vi "电导率_所有参数读取.vi"(8 "error in (no error)":errorcluster caption="错误输入（无错误）", 11 "MB session in":refnum<class "MB_Master.lvclass">) -> (0 "error out":errorcluster caption="错误输出", 2 "输出值":T1 {"电极型号标志" items=["NULL", "pH", "Cond", "DO", "Turb"]; "电极状态标志" items=["OK"]}, 3 "MB session out":refnum<class "MB_Master.lvclass">)   [LabVIEW 2016, in "斯坦道多参数.lvlib"]
uses:
  <vilib>/Plasmionique/MB Master/MB_Master/MB_Master.lvclass
  <vilib>/Plasmionique/MB Master/MB Master.lvlib
  <vilib>/ptbypt/NI_PtbyPt.lvlib
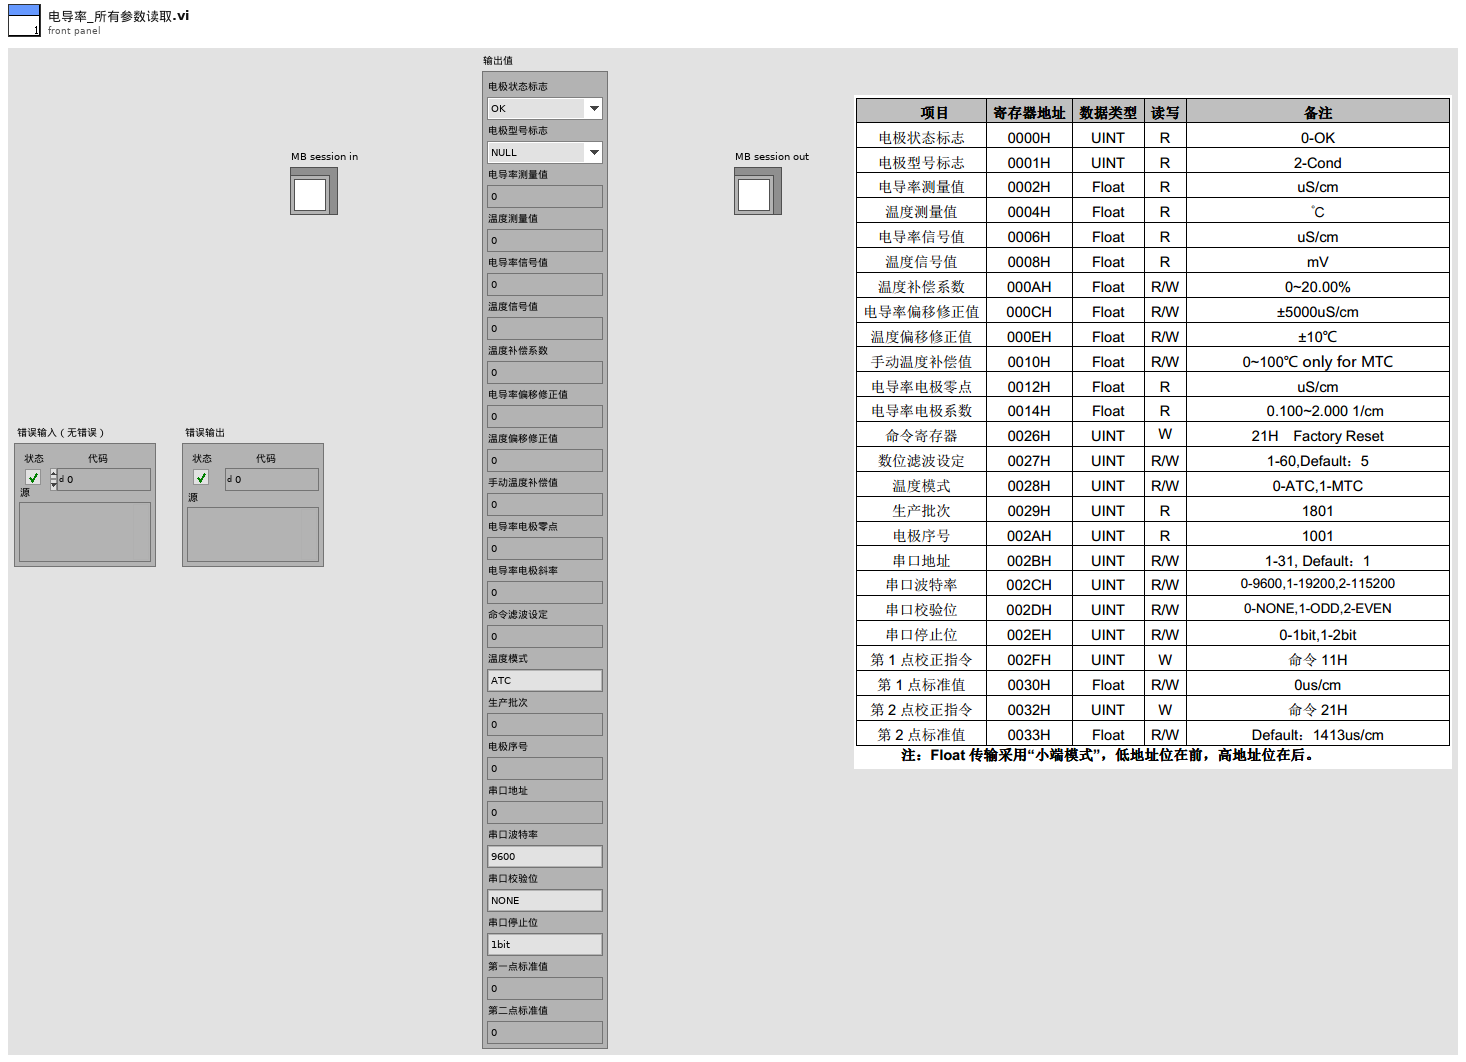
[diagram p1: front panel]
types:
  T1 = cluster{"电极状态标志":u16, "电极型号标志":u16, "电导率测量值":sgl, "温度测量值":sgl, "电导率信号值":sgl, "温度信号值":sgl, "温度补偿系数":sgl, "电导率偏移修正值":sgl, "温度偏移修正值":sgl, "手动温度补偿值":sgl, "电导率电极零点":sgl, "电导率电极斜率":sgl, "命令滤波设定":u16, "温度模式":enum16{"ATC", "MTC"}, "生产批次":u16, "电极序号":u16, "串口地址":u16, "串口波特率":enum16{"9600", "19200", "115200"}, "串口校验位":enum16{"NONE", "ODD", "EVEN"}, "串口停止位":enum16{"1bit", "2bit"}, "第一点标准值":sgl, "第二点标准值":sgl}
  T2 = cluster{u16, u16, "Filtered x":dbl, "数值":sgl, "数值":sgl, "数值":sgl, "数值":sgl, "数值":sgl, "数值":sgl, "数值":sgl, "数值":sgl, "数值":sgl, u16, u16, u16, u16, u16, u16, u16, u16, "数值":sgl, "数值":sgl}
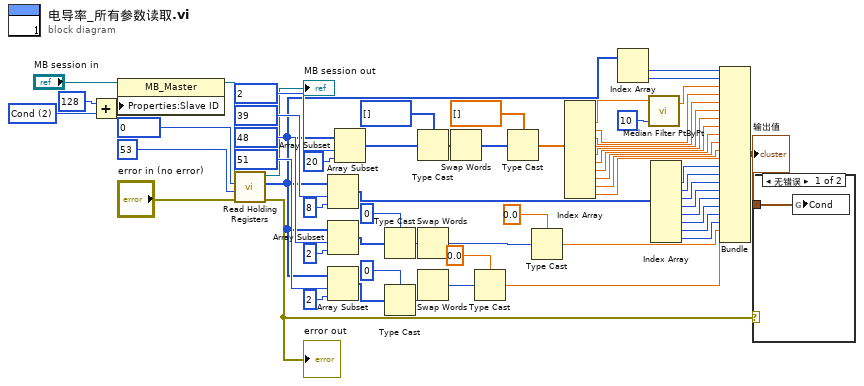
[diagram p0: block diagram]
diagram:
  w61 = u16 2 items=["NULL", "pH", "Cond", "DO", "Turb"] ("数值")
  n1 = Add(x=u16 128, y=w61) -> (x+y=w60:u16)
  n2 = property class="MB_Master"(reference="MB session in", "Properties:Slave ID"=w60) -> (reference out=w14:refnum<class "MB_Master.lvclass">)  [unwired: 1 in, 1 out]
  n3 = call <vilib>:"Read Holding Registers.vi"("error in (no error)"="error in (no error)", "quantity"=u16 53, "starting address"=u16 0, "MB session in"=w14) -> ("error out"=w7:errorcluster, "Registers"=w28:u16[], "MB session out"=→"MB session out":refnum<class "MB_Master.lvclass">)  [unwired: 5 in]
  "error out" <- w7
  n4 = Array Subset(array=w28, index=u16 39 ("starting address"), length=8 ("长度")) -> (w41:u16[])
  n5 = Array Subset(array=w28, index=u16 48 ("starting address"), length=2 ("长度")) -> (w23:u16[])
  n6 = Array Subset(array=w28, index=u16 51 ("starting address"), length=2 ("长度")) -> (w18:u16[])
  n7 = Array Subset(array=w28, index=u16 2 ("starting address"), length=20 ("长度")) -> (w49:u16[])
  n8 = Type Cast(type=u32 0 ("数值"), x=w23) -> (*(type *) &x=w26:u32)
  n9 = Type Cast(type=u32 0 ("数值"), x=w18) -> (*(type *) &x=w20:u32)
  n10 = Type Cast(type=u32[] [] ("数组 2"), x=w49) -> (*(type *) &x=w51:u32[])
  n11 = Swap Words(1:w26) -> (0:w27:u32)
  n12 = Swap Words(1:w20) -> (0:w19:u32)
  n13 = Swap Words(1:w51) -> (0:w53:u32[])
  n14 = Type Cast(type=sgl 0.0 ("数值"), x=w19) -> (*(type *) &x=w16:sgl)
  n15 = Type Cast(type=sgl[] [] ("数组 2"), x=w53) -> (*(type *) &x=w48:sgl[])
  n16 = Type Cast(type=sgl 0.0 ("数值"), x=w27) -> (*(type *) &x=w17:sgl)
  n17 = Index Array(array=w48) -> (element #1=w2:sgl, element #2=w47:sgl, element #3=w46:sgl, element #4=w45:sgl, element #5=w13:sgl, element #6=w12:sgl, element #7=w11:sgl, element #8=w10:sgl, element #9=w9:sgl, element #10=w8:sgl)  [unwired: 10 in]
  n18 = Index Array(array=w28) -> (element #1=w56:u16, element #2=w55:u16)  [unwired: 2 in]
  n19 = call <vilib>:"Median Filter PtByPt.vi"("rank"=10, "x"=w2) -> ("Filtered x"=w1:dbl)  [unwired: 2 in, 1 out]
  n20 = Index Array(array=w41) -> (element #1=w40:u16, element #2=w39:u16, element #3=w38:u16, element #4=w37:u16, element #5=w36:u16, element #6=w35:u16, element #7=w34:u16, element #8=w33:u16)  [unwired: 8 in]
  n21 = Bundle(w56, w55, "Filtered x"=w1, "数值"=w47, "数值"=w46, "数值"=w45, "数值"=w13, "数值"=w12, "数值"=w11, "数值"=w10, "数值"=w9, "数值"=w8, w40, w39, w38, w37, w36, w35, w34, w33, "数值"=w17, "数值"=w16) -> (w6:T2)  [unwired: 1 in]
  "输出值" <- w6
  n22 = case shown="无错误" w7 {
    tunnel: w6 -> [w62 _]
    frame No Error {
      n23 = global write "国弘过程全局变量.vi" "Cond"(w62) -> ()
    }
    frame Error {
    }
  }
